vi "Lakeshore Gaussmeter.vi"(8 "error in (no error)":errorcluster, 11 "Lakeshore Gaussmeter in":refnum<class "Lakeshore Gaussmeter.lvclass">) -> (0 "error out":errorcluster, 3 "Lakeshore Gaussmeter out":refnum<class "Lakeshore Gaussmeter.lvclass">)   [LabVIEW 2017, in "Lakeshore Gaussmeter.lvclass"]
uses:
  Lakeshore Gaussmeter.lvclass
  Global/GPIB Numbers.vi
panel:
  out "Status":string
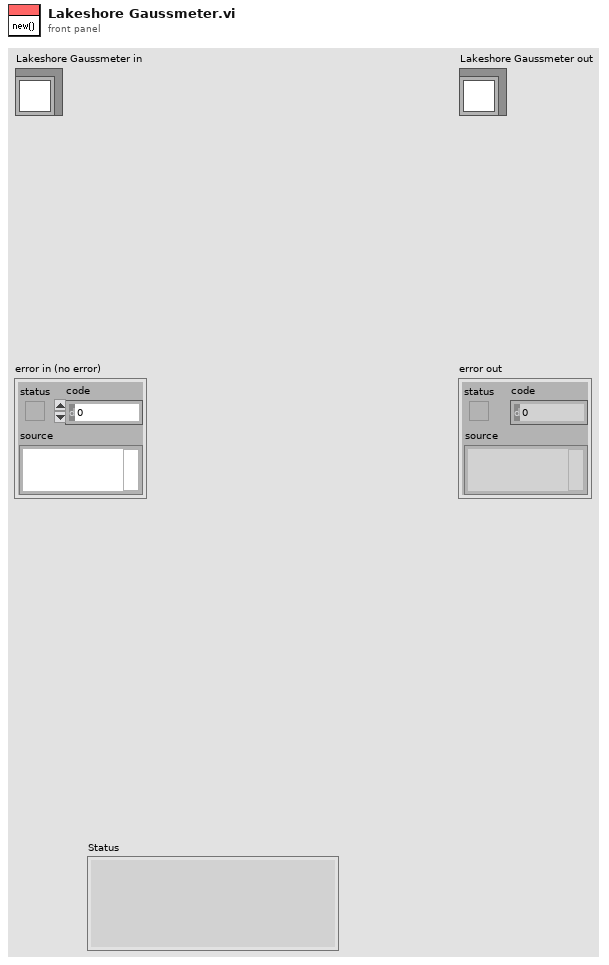
[diagram p1: front panel]
types:
  T1 = typedef "GPIB Type Def.ctl" = cluster{"Name":string, "bus":dbl, "GPIB":dbl, "GPIB as string":string, "byte":i32, "VISA Resource Name":refnum<visa-resource-name>}
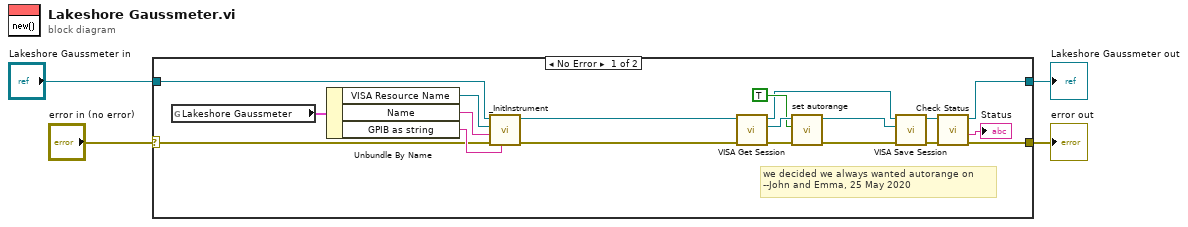
[diagram p0: block diagram]
diagram:
  n1 = case shown="No Error" "error in (no error)" {
    selector: "error in (no error)" -> [w18 w25]
    tunnel: [w15 w25] -> w3
    tunnel: [w16 w24] -> w1
    tunnel: "Lakeshore Gaussmeter in" -> [w19 w24]
    frame No Error {
      # "we decided we always wanted autorange on\n--John and Emma, 25 May 2020"
      n2 = global read "GPIB Numbers.vi" "Lakeshore Gaussmeter"() -> (w23:T1)
      n3 = Unbundle By Name(w23) -> ("VISA Resource Name"=w22:refnum<visa-resource-name>, "Name"=w21:string, "GPIB as string"=w20:string)
      n4 = call-dynamic "_InitInstrument.vi"("GPIB as string"=w20, "error in (no error)"=w18, "Name"=w21, "VISA Resource Name"=w22, "Instrument in"=w19) -> ("error out"=w8:errorcluster, "Instrument out"=w9:refnum<class "Lakeshore Gaussmeter.lvclass">)  [unwired: 1 in, 4 out]
      n5 = call-dynamic "VISA Get Session.vi"("error in (no error)"=w8, "Instrument.lvclass in"=w9) -> ("error out"=w13:errorcluster, "VISA Resource Name"=w11:refnum<visa-resource-name>, "Instrument.lvclass out"=w5:refnum<class "Lakeshore Gaussmeter.lvclass">)  [unwired: 7 out]
      n6 = call "set autorange.vi"("error in (no error)"=w13, "Auto Range (F: Off)"=TRUE, "VISA session"=w11) -> ("error out"=w14:errorcluster, "dup VISA session"=w12:refnum<visa-resource-name>)  [unwired: 7 in]
      n7 = call-dynamic "VISA Save Session.vi"("error in (no error)"=w14, "VISA Resource Name"=w12, "Instrument.lvclass in"=w5) -> ("error out"=w7:errorcluster, "Instrument.lvclass out"=w6:refnum<class "Lakeshore Gaussmeter.lvclass">)  [unwired: 7 out]
      n8 = call-dynamic "Check Status.vi"("error in (no error)"=w7, "Lakeshore Gaussmeter in"=w6) -> ("error out"=w15:errorcluster, "Status"=→"Status":string, "Lakeshore Gaussmeter out"=w16:refnum<class "Lakeshore Gaussmeter.lvclass">)  [unwired: 6 in, 1 out]
    }
    frame Error {
    }
  }
  "error out" <- w3
  "Lakeshore Gaussmeter out" <- w1
